vi "ATSh_SetRecordCount.vi"(8 "NoLimit (T)":bool=TRUE, 10 "#Record":u32=1, 11 "HandleIn":u32) -> (0 "Return Code":u32, 3 "HandleOut":u32)   [LabVIEW 2014]
doc: "_____AlazarTech, Scope_____\n\nConfigure the number of records for the device to capture."
uses:
  ATSApi.dll
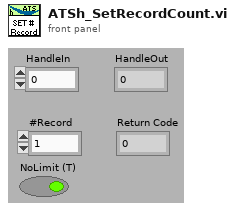
[diagram p1: front panel]
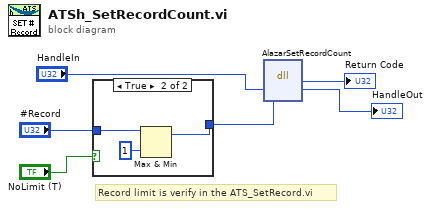
[diagram p0: block diagram]
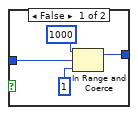
[diagram p2: hidden frame]
diagram:
  # "Record limit is verify in the ATS_SetRecord.vi"
  n1 = case shown="True" "NoLimit (T)" {
    tunnel: "#Record" -> [w10 w13]
    tunnel: [w7 w12] -> w2
    frame False {
      n2 = In Range and Coerce(upper limit=u32 1000, x=w10, lower limit=u32 1) -> (coerced(x)=w7:u32)  [unwired: 1 out]
    }
    frame True {
      n3 = Max & Min(x=w13, y=u32 1) -> (max(x,y)=w12:u32)  [unwired: 1 out]
    }
  }
  n4 = dll-call lib="D:/IntensityOCT/trunk/ATSApi.dll" fn="AlazarSetRecordCount"("h"="HandleIn", "Count"=w2) -> (→"Return Code":u32, "h"=→"HandleOut":u32)  [unwired: 4 in, 2 out]
